vi "gen_tooth_function.vi"(8 "error in (no error)":errorcluster, 10 "z signal graph ref":refnum<vi>, 11 "TrajectoryAK101022Resonance in":refnum<class "TrajectoryAK101022Resonance.lvclass">) -> (0 "error out":errorcluster, 1 "z-frequency":dbl[unit], 2 "z points":dbl[unit][](array[numeric]), 3 "TrajectoryAK101022Resonance out":refnum<class "TrajectoryAK101022Resonance.lvclass">)   [LabVIEW 2010, in "TrajectoryAK101022Resonance.lvclass"]
uses:
  TrajectoryAK101022Resonance.lvclass
  FPGAWrapper/FPGAWrapperAK101022Resonance/FPGAWrapperAK101022Resonance/FPGAWrapperAK101022Resonance.lvclass
  TrajectoryAK101022Resonance.lvclass/TrajectoryAK101022Resonance.ctl
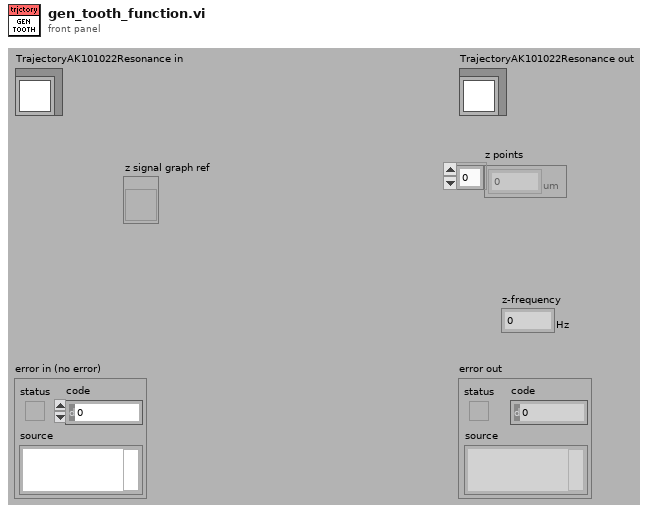
[diagram p1: front panel]
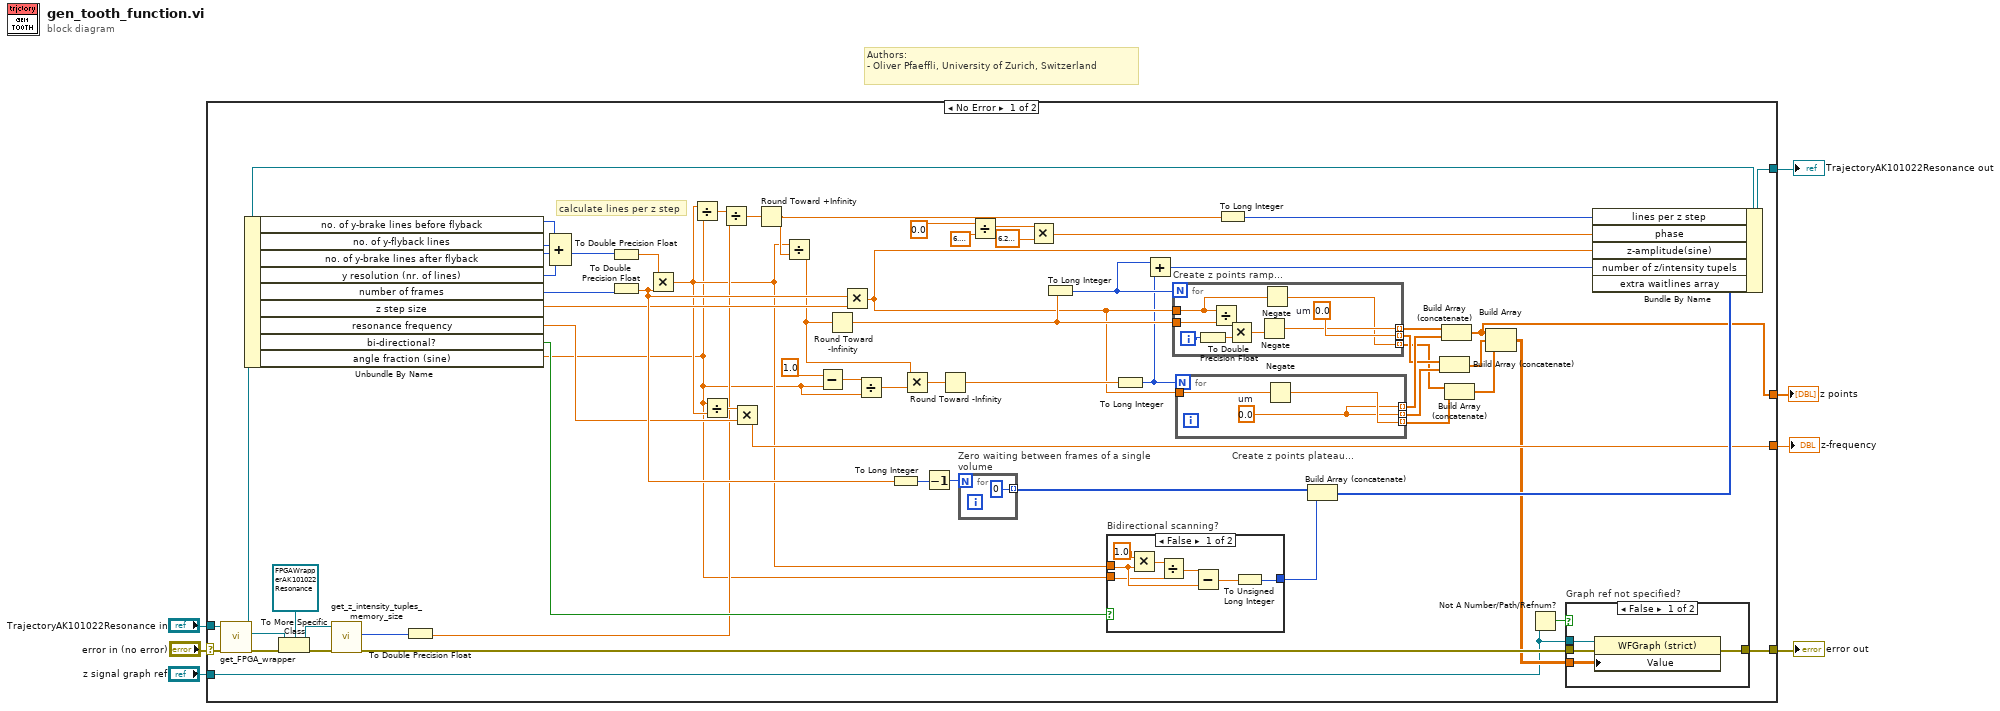
[diagram p0: block diagram]
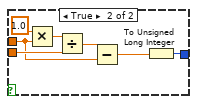
[diagram p3: hidden frame]
diagram:
  # "Authors: \n- Oliver Pfaeffli, University of Zurich, Switzerland"
  n1 = case shown="No Error" "error in (no error)" {
    selector: "error in (no error)" -> [w58 w106]
    tunnel: [w33 w106] -> w6
    tunnel: [w72 w105] -> w5
    tunnel: "TrajectoryAK101022Resonance in" -> [w57 w105]
    tunnel: [w35 _] -> w3
    tunnel: "z signal graph ref" -> [w31 _]
    tunnel: [w11 _] -> w1
    frame No Error {
      # "calculate lines per z step"
      n2 = call-dynamic "get_FPGA_wrapper.vi"("error in (no error)"=w58, "TrajectoryMG100122GenericFPGA in"=w57) -> ("error out"=w54:errorcluster, "GenericFPGAWrapper.lvclass"=w55:refnum<class "GenericFPGAWrapper.lvclass">, "TrajectoryMG100122GenericFPGA out"=w56:refnum<class "TrajectoryAK101022Resonance.lvclass">)  [unwired: 7 in]
      n3 = Unbundle By Name(w56) -> ("no. of y-brake lines before flyback"=w62:i32, "no. of y-flyback lines"=w61:i32, "no. of y-brake lines after flyback"=w60:i32, "y resolution (nr. of lines)"=w41:i32, "number of frames"=w39:i32, "z step size"=w38:dbl[unit], "resonance frequency"=w42:dbl[unit], "bi-directional?"=w47:bool, "angle fraction (sine)"=w25:dbl)
      n4 = To More Specific Class(target class=refnum<class "FPGAWrapperAK101022Resonance.lvclass"> refnum ("FPGAWrapperAK101022Resonance.lvclass"), reference=w55, error in=w54) -> (specific class reference=w51:refnum<class "FPGAWrapperAK101022Resonance.lvclass">, error out=w53:errorcluster)
      n5 = call "get_z_intensity_tuples_memory_size.vi"("error in (no error)"=w53, "FPGAWrapperAK101022Resonance in"=w51) -> ("error out"=w34:errorcluster, "z/intensity memory size"=w50:i32)  [unwired: 7 in, 1 out]
      n6 = To Double Precision Float(number=w50) -> (double precision float=w37:dbl)
      n7 = Compound Arithmetic op=ADD(w62, w61, w60, w41) -> (w40:i32)
      n8 = To Double Precision Float(number=w40) -> (double precision float=w67:dbl)
      n9 = To Double Precision Float(number=w39) -> (double precision float=w49:dbl)
      n10 = Multiply(x=w67, y=w49) -> (x*y=w29:dbl)
      n11 = Divide(x=w29, y=w25) -> (x/y=w64:dbl)
      n12 = Divide(x=w25, y=w29) -> (x/y=w59:dbl)
      n13 = Divide(x=w64, y=w37) -> (x/y=w66:dbl)
      n14 = Multiply(x=w59, y=w42) -> (x*y=w35:dbl[unit])
      n15 = Round Toward +Infinity(x=w66) -> (ceil(x): smallest int >= x=w63:dbl)
      n16 = Divide(x=w29, y=w63) -> (x/y=w23:dbl)
      n17 = Subtract(x=1.0, y=w25) -> (x-y=w26:dbl)
      n18 = Round Toward -Infinity(1:w23) -> (0:w44:dbl)
      n19 = Multiply(x=w49, y=w38) -> (x*y=w20:dbl[unit])
      n20 = Divide(x=w26, y=w25) -> (x/y=w24:dbl)
      n21 = To Long Integer(number=w49) -> (32bit integer=w46:i32)
      n22 = Multiply(x=w23, y=w24) -> (x*y=w22:dbl)
      n23 = Decrement(x=w46) -> (x-1=w45:i32)
      n24 = Round Toward -Infinity(1:w22) -> (0:w21:dbl)
      n25 = for "Zero waiting between frames of a single volume" {
        N: w45 -> [_]
        tunnel: [u32 0] -> w48 mode=indexing
      }
      n26 = Divide(x=0.0, y=6.283185307179586) -> (x/y=w69:dbl)
      n27 = Multiply(x=w69, y=dbl[unit] 6.283185307179586) -> (x*y=w68:dbl[unit])
      n28 = To Long Integer(number=w44) -> (32bit integer=w10:i32)
      n29 = case "Bidirectional scanning?" shown="False" w47 {
        tunnel: w29 -> [w83 w89]
        tunnel: [w81 w94] -> w43
        tunnel: w25 -> [w82 w91]
        frame False {
          n30 = Multiply(x=1.0, y=w83) -> (x*y=w86:dbl)
          n31 = Divide(x=w86, y=w82) -> (x/y=w85:dbl)
          n32 = Subtract(x=w85, y=w83) -> (x-y=w84:dbl)
          n33 = To Unsigned Long Integer(number=w84) -> (unsigned 32bit integer=w81:u32)
        }
        frame True {
          n34 = Multiply(x=1.0, y=w89) -> (x*y=w92:dbl)
          n35 = Divide(x=w92, y=w91) -> (x/y=w90:dbl)
          n36 = Subtract(x=w90, y=w89) -> (x-y=w88:dbl)
          n37 = To Unsigned Long Integer(number=w88) -> (unsigned 32bit integer=w94:u32)
        }
      }
      n38 = To Long Integer(number=w21) -> (32bit integer=w9:i32)
      n39 = Add(x=w10, y=w9) -> (x+y=w8:i32)
      n40 = for "Create z points ramp..." {
        N: w10 -> [_]
        tunnel: w44 -> [w103]
        tunnel: w20 -> [w97]
        tunnel: [w98] -> w19 mode=indexing
        tunnel: [w99] -> w17 mode=indexing
        tunnel: [w96] -> w14 mode=indexing
        i -> [w104]
        w99 = dbl[unit] 0.0  # um
        n41 = To Double Precision Float(number=w104) -> (double precision float=w102:dbl)
        n42 = Divide(x=w97, y=w103) -> (x/y=w101:dbl[unit])
        n43 = Multiply(x=w101, y=w102) -> (x*y=w100:dbl[unit])
        n44 = Negate(x=w100) -> (-x=w98:dbl[unit])
        n45 = Negate(x=w97) -> (-x=w96:dbl[unit])
      }
      n46 = for "Create z points plateau..." {
        N: w9 -> [_]
        tunnel: w20 -> [w75]
        tunnel: [w73] -> w16 mode=indexing
        tunnel: [w74] -> w13 mode=indexing
        tunnel: [w73] -> w18 mode=indexing
        w73 = dbl[unit] 0.0  # um
        n47 = Negate(x=w75) -> (-x=w74:dbl[unit])
      }
      n48 = To Long Integer(number=w63) -> (32bit integer=w65:i32)
      n49 = Build Array (concatenate)(w48, w43) -> (w36:u32[])
      n50 = Build Array (concatenate)(w17, w16) -> (w15:dbl[unit][])
      n51 = Build Array (concatenate)(w19, w18) -> (w11:dbl[unit][])
      n52 = Build Array (concatenate)(w14, w13) -> (w12:dbl[unit][])
      n53 = Build Array(w11, w15, w12) -> (w32:dbl[unit][][])
      n54 = Not A Number/Path/Refnum?(number/path/refnum=w31) -> (NaN/Path/Refnum?=w30:bool)
      n55 = case "Graph ref not specified?" shown="False" w30 {
        tunnel: w34 -> [w79 w80]
        tunnel: [w78 w80] -> w33
        tunnel: w31 -> [w77 _]
        tunnel: w32 -> [w76 _]
        frame False {
          n56 = property class="WFGraph (strict)"(reference=w77, error in=w79, "Value"=w76) -> (error out=w78:errorcluster)  [unwired: 1 out]
        }
        frame True {
        }
      }
      n57 = Bundle By Name(cluster=w56, "lines per z step"=w65, "phase"=w68, "z-amplitude(sine)"=w20, "number of z/intensity tupels"=w8, "extra waitlines array"=w36) -> (w72:refnum<class "TrajectoryAK101022Resonance.lvclass">)
    }
    frame Error {
    }
  }
  "error out" <- w6
  "TrajectoryAK101022Resonance out" <- w5
  "z-frequency" <- w3
  "z points" <- w1
